vi "Poll Containers.vi"(8 "error in (no error)":errorcluster, 11 "Storage Line in":refnum<class "Storage Line.lvclass">) -> ()   [LabVIEW 2015, in "cRIO-Carbondioxide.lvlib" / "CO2-Actor.lvlib" / "Storage Line.lvclass"]
uses:
  Storage Line.lvclass
  CO2 Actor/CO2 Actor.lvclass
  Storage Line.lvclass/Storage Line.ctl
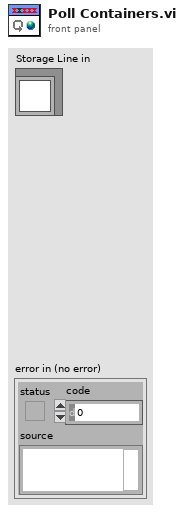
[diagram p1: front panel]
types:
  T1 = typedef "Sample Container.ctl" = cluster{"Sample In":refnum<k21>, "Sample Name":refnum<k21>, "Ti Cathode":refnum<k21>, "SampleQ":refnum<queue>}
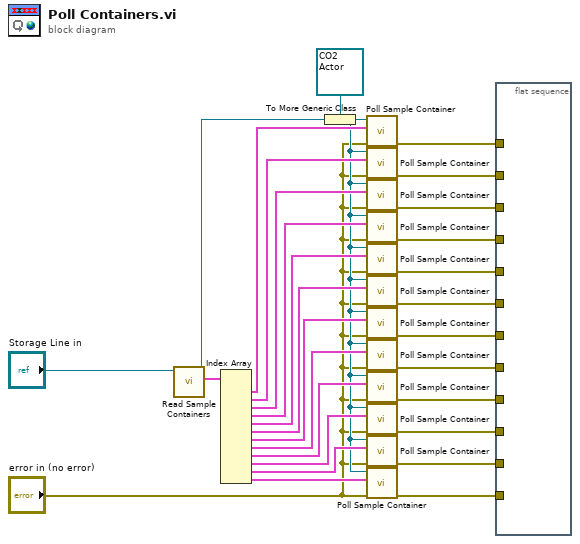
[diagram p0: block diagram]
diagram:
  n1 = call "Read Sample Containers.vi"("Storage Line in"="Storage Line in") -> ("Sample Containers"=w28:T1[], "Storage Line out"=w29:refnum<class "Storage Line.lvclass">)  [unwired: 9 in]
  n2 = Index Array(array=w28) -> (element #1=w27:T1, element #2=w25:T1, element #3=w24:T1, element #4=w23:T1, element #5=w22:T1, element #6=w21:T1, element #7=w20:T1, element #8=w19:T1, element #9=w18:T1, element #10=w17:T1, element #11=w16:T1, element #12=w26:T1)  [unwired: 12 in]
  n3 = To More Generic Class(target class=refnum<class "CO2 Actor.lvclass"> refnum ("CO2 Actor in"), reference=w29) -> (generic class reference=w15:refnum<class "CO2 Actor.lvclass">)
  n4 = call-dynamic "Poll Sample Container.vi"("error in (no error)"="error in (no error)", "Sample Container"=w27, "CO2 Actor in"=w15) -> ("error out"=w2:errorcluster)  [unwired: 8 in]
  n5 = call-dynamic "Poll Sample Container.vi"("error in (no error)"="error in (no error)", "Sample Container"=w25, "CO2 Actor in"=w15) -> ("error out"=w3:errorcluster)  [unwired: 8 in]
  n6 = call-dynamic "Poll Sample Container.vi"("error in (no error)"="error in (no error)", "Sample Container"=w24, "CO2 Actor in"=w15) -> ("error out"=w4:errorcluster)  [unwired: 8 in]
  n7 = call-dynamic "Poll Sample Container.vi"("error in (no error)"="error in (no error)", "Sample Container"=w23, "CO2 Actor in"=w15) -> ("error out"=w5:errorcluster)  [unwired: 8 in]
  n8 = call-dynamic "Poll Sample Container.vi"("error in (no error)"="error in (no error)", "Sample Container"=w22, "CO2 Actor in"=w15) -> ("error out"=w6:errorcluster)  [unwired: 8 in]
  n9 = call-dynamic "Poll Sample Container.vi"("error in (no error)"="error in (no error)", "Sample Container"=w21, "CO2 Actor in"=w15) -> ("error out"=w7:errorcluster)  [unwired: 8 in]
  n10 = call-dynamic "Poll Sample Container.vi"("error in (no error)"="error in (no error)", "Sample Container"=w20, "CO2 Actor in"=w15) -> ("error out"=w8:errorcluster)  [unwired: 8 in]
  n11 = call-dynamic "Poll Sample Container.vi"("error in (no error)"="error in (no error)", "Sample Container"=w19, "CO2 Actor in"=w15) -> ("error out"=w9:errorcluster)  [unwired: 8 in]
  n12 = call-dynamic "Poll Sample Container.vi"("error in (no error)"="error in (no error)", "Sample Container"=w18, "CO2 Actor in"=w15) -> ("error out"=w10:errorcluster)  [unwired: 8 in]
  n13 = call-dynamic "Poll Sample Container.vi"("error in (no error)"="error in (no error)", "Sample Container"=w17, "CO2 Actor in"=w15) -> ("error out"=w11:errorcluster)  [unwired: 8 in]
  n14 = call-dynamic "Poll Sample Container.vi"("error in (no error)"="error in (no error)", "Sample Container"=w16, "CO2 Actor in"=w15) -> ("error out"=w12:errorcluster)  [unwired: 8 in]
  n15 = call-dynamic "Poll Sample Container.vi"("error in (no error)"="error in (no error)", "Sample Container"=w26, "CO2 Actor in"=w15) -> ("error out"=w13:errorcluster)  [unwired: 8 in]
  n16 = flat-sequence {
    tunnel: w13 -> [_]
    tunnel: w12 -> [_]
    tunnel: w11 -> [_]
    tunnel: w10 -> [_]
    tunnel: w9 -> [_]
    tunnel: w8 -> [_]
    tunnel: w7 -> [_]
    tunnel: w6 -> [_]
    tunnel: w5 -> [_]
    tunnel: w4 -> [_]
    tunnel: w3 -> [_]
    tunnel: w2 -> [_]
    frame #0 {
    }
  }
